vi "Controller Write FXP16.5.vi"(3 "Error In":errorcluster, 4 "Values":fxp<+/-,16,5>[](array[numeric]), 5 "Variables":refnum<k21>[](array[refnum])) -> (0 "Error Out":errorcluster)   [LabVIEW 2011, in "Controller VIs.lvlib"]
uses:
  Controller VIs.lvlib
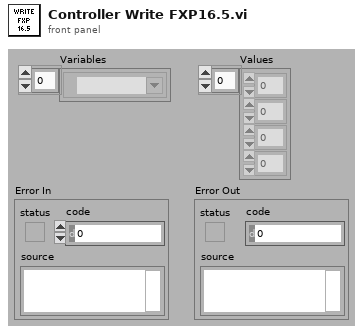
[diagram p1: front panel]
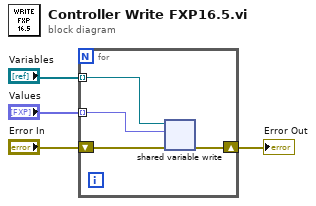
[diagram p0: block diagram]
diagram:
  n1 = for {
    tunnel: "Values" -> [w8] mode=indexing
    tunnel: "Variables" -> [w7] mode=indexing
    shift-right: [w5] -> w3
    shift-left: "Error In" -> [w6]
    n2 = shared-variable-write(w7, w6, w8) -> (w5:errorcluster)  [unwired: 1 out]
  }
  "Error Out" <- w3
